vi "MAUI.GetPrivateEvents.vi"(8 "error in (no error)":errorcluster, 11 "MAUI":refnum<class "MAUI.lvclass">) -> (0 "error out":errorcluster, 2 "Private Events":T1, 3 "MAUI out":refnum<class "MAUI.lvclass">)   [LabVIEW 2016, in "MAUI.lvclass"]
doc: "---------------------------------------------------------------\nJKI State Machine Objects™\nhttp://jki.net/state-machine-objects/\nCopyright (C) 2005-2015, JKI <info@jki.net>\nALL RIGHTS RESERVEDJKI State Machine Objects (SMO) 1.0.0.4\nJKI - JKI\nCopyright (c) 2015, JKI"
uses:
  MAUI.lvclass
  Typedefs/PrivateEvents--Cluster.ctl
  Typedefs/PrivateEvents--MAUI.SetLeftData.ctl
  Typedefs/PrivateEvents--MAUI.SetRightData.ctl
  Typedefs/PrivateEvents--MAUI.GetRightData.ctl
  Typedefs/PanelData.ctl
  Typedefs/PrivateEvents--MAUI.GetLeftData.ctl
  Typedefs/PanelDataNotifier.ctl
  Typedefs/PrivateEvents--MAUI.SetEmbedded.ctl
  <vilib>/Levylab/Embedded SMO UI/EmbeddedSMO.lvclass
  Typedefs/PrivateEvents--MAUI.GetEmbedded.ctl
  Typedefs/PrivateEvents--MAUI.Update Left Subpanel.ctl
  Typedefs/PrivateEvents--MAUI.UpdateRightSubpanel.ctl
  MAUI.lvclass/MAUI.ctl
panel:
  # "For instructions on how to use the JKI State Machine Objects, examples and video tutorials, visit:\nhttp://jki.net/state-machine-objects/\n\nJKI State Machine Objects™\nhttp://jki.net/state-machine-objects/\nCopyright (C) 2005-2015, JKI <info@jki.net>\nALL RIGHTS RESERVED"
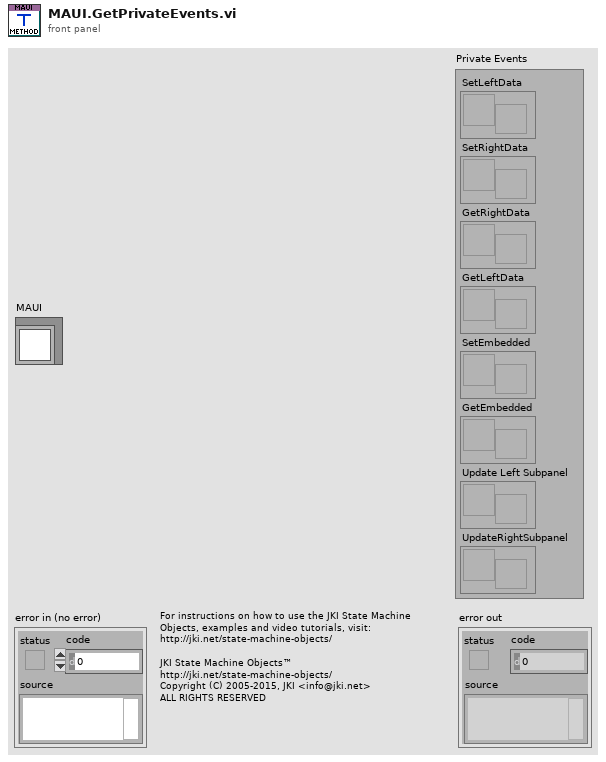
[diagram p1: front panel]
types:
  T1 = typedef "MAUI.lvclass/PrivateEvents--Cluster.ctl" = cluster{"SetLeftData":refnum<user-event>, "SetRightData":refnum<user-event>, "GetRightData":refnum<user-event>, "GetLeftData":refnum<user-event>, "SetEmbedded":refnum<user-event>, "GetEmbedded":refnum<user-event>, "Update Left Subpanel":refnum<user-event>, "UpdateRightSubpanel":refnum<user-event>}
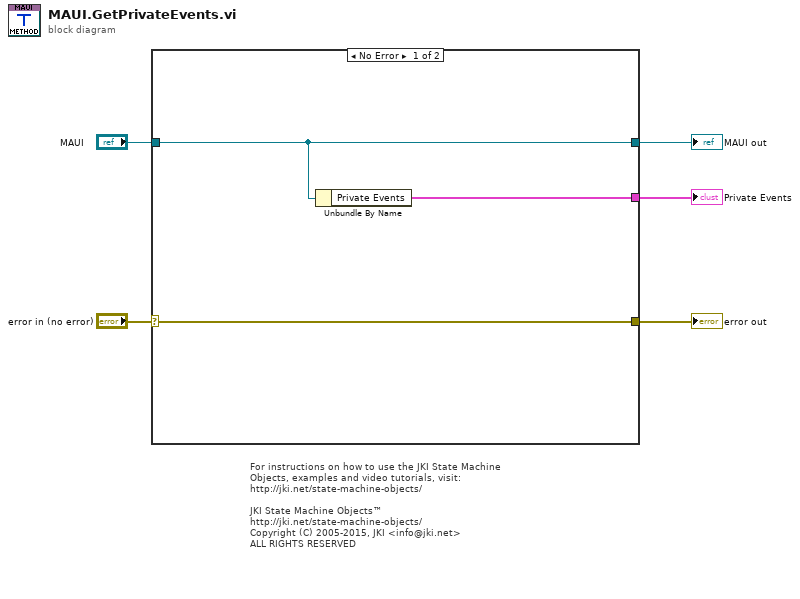
[diagram p0: block diagram]
diagram:
  # "For instructions on how to use the JKI State Machine Objects, examples and video tutorials, visit:\nhttp://jki.net/state-machine-objects/\n\nJKI State Machine Objects™\nhttp://jki.net/state-machine-objects/\nCopyright (C) 2005-2015, JKI <info@jki.net>\nALL RIGHTS RESERVED"
  n1 = case shown="No Error" "error in (no error)" {
    selector: "error in (no error)" -> [w8 w9]
    tunnel: "MAUI" -> [w7 w10]
    tunnel: [w8 w9] -> w4
    tunnel: [w7 w10] -> w3
    tunnel: [w6 _] -> w1
    frame No Error {
      n2 = Unbundle By Name(w7) -> ("Private Events"=w6:T1)
    }
    frame Error {
    }
  }
  "error out" <- w4
  "MAUI out" <- w3
  "Private Events" <- w1
